vi "Identify.vi"(8 "error in (no error)":errorcluster, 11 "NI Generic Parser in":refnum<class "NI Generic Parser.lvclass">) -> (0 "error out":errorcluster, 2 "Plugin is Valid":bool, 3 "NI Generic Parser out":refnum<class "NI Generic Parser.lvclass">)   [LabVIEW 2016, in "NI Generic Parser.lvlib" / "NI Generic Parser.lvclass"]
uses:
  NI Generic Parser.lvclass
  C:/Sequence Automation/Plugins/File Parsing Interface.lvlibp/File Parsing Interface.lvclass
  Plugins/File Parsing Interface.lvlibp/Accessors/File to Parse/Read File to Parse.vi
  <vilib>/addons/_office/excel.llb/Excel Get Data ([str]).vi
  <vilib>/Utility/NIReport.llb/NI_report.lvclass
  <vilib>/Utility/NIReport.llb/Excel/NI_Excel.lvclass
  <vilib>/addons/_office/NI_ReportGenerationToolkit.lvlib
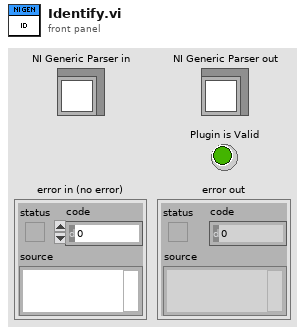
[diagram p1: front panel]
types:
  T1 = enum16{"Standard Report", "HTML", "Word", "Excel"}
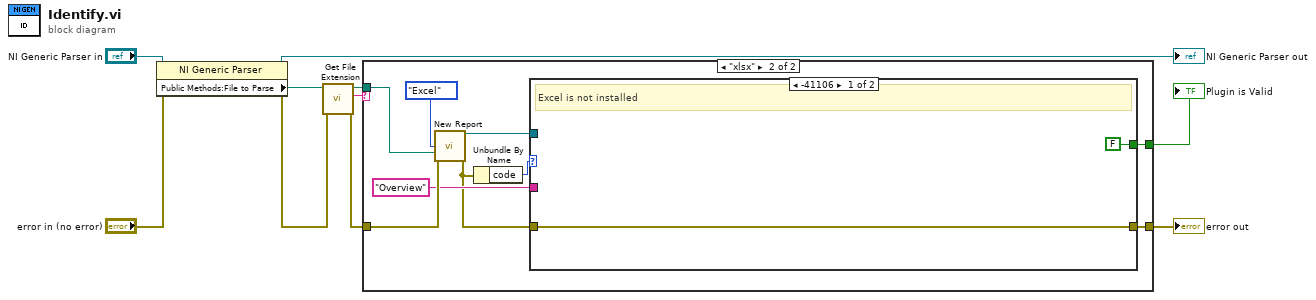
[diagram p0: block diagram]
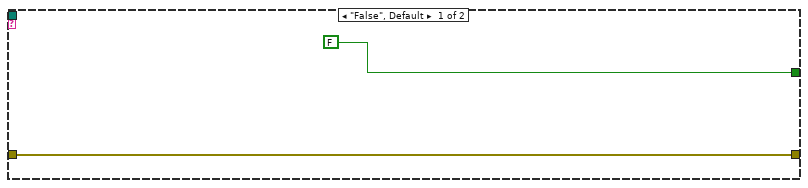
[diagram p2: hidden frame]
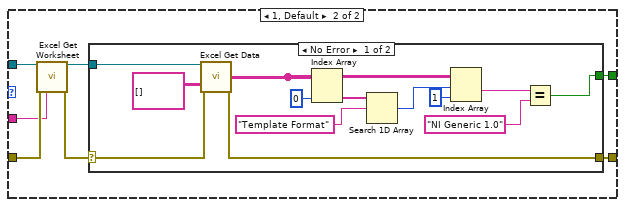
[diagram p3: hidden frame]
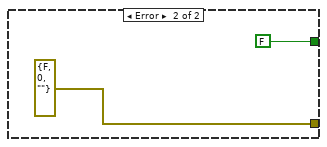
[diagram p4: hidden frame]
diagram:
  n1 = property class="NI Generic Parser"(reference="NI Generic Parser in", error in="error in (no error)") -> (reference out=→"NI Generic Parser out":refnum<class "NI Generic Parser.lvclass">, error out=w7:errorcluster, "Public Methods:File to Parse"=w6:path)
  n2 = call <vilib>:"Get File Extension.vi"("error in (no error)"=w7, "file"=w6) -> ("error out"=w4:errorcluster, "lowercase file extension"=w5:string, "dup file"=w2:path)  [unwired: 5 in, 2 out]
  n3 = case shown="\"xlsx\"" w5 {
    tunnel: w4 -> [w11 w19]
    tunnel: [FALSE w15] -> w3
    tunnel: w2 -> [_ w21]
    tunnel: [w11 w16] -> w1
    frame "False", Default {
    }
    frame "xlsx" {
      n4 = call <vilib>:"New Report.vi"("report type"=T1."Excel", "template (empty)"=w21, "error in (no error)"=w19) -> ("report out"=w18:refnum<class "NI_report.lvclass">, "error out"=w14:errorcluster)  [unwired: 11 in]
      n5 = Unbundle By Name(w14) -> ("code"=w13:i32)
      n6 = case shown="-41106" w13 {
        tunnel: w18 -> [_ w30]
        tunnel: w14 -> [w23 w29]
        tunnel: "Overview" ("name (\"\")") -> [_ w28]
        tunnel: [w23 w25] -> w16
        tunnel: [FALSE w24] -> w15
        frame -41106 {
          # "Excel is not installed"
        }
        frame 1, Default {
          n7 = call <vilib>:"Excel Get Worksheet.vi"("report in"=w30, "error in (no error)"=w29, "name (\"\")"=w28) -> ("report out"=w27:refnum<class "NI_report.lvclass">, "error out"=w26:errorcluster)  [unwired: 11 in]
          n8 = case shown="No Error" w26 {
            selector: w26 -> [w42 _]
            tunnel: w27 -> [w43 _]
            tunnel: [w40 errorcluster {"status"=FALSE, "code"=0, "source"=""} ("error out")] -> w25
            tunnel: [w31 FALSE] -> w24
            frame No Error {
              n9 = call-poly <vilib>:"Excel Get Data.vi"("report in"=w43, "data type"=string[][] [], "error in (no error)"=w42) -> ("data"=w36:string[][], "error out"=w40:errorcluster)  [unwired: 10 in, 1 out]
              n10 = Index Array(array=w36, index (col)=0 ("disabled index (col)")) -> (element=w38:string[])  [unwired: 1 in]
              n11 = Search 1D Array(1D array=w38, element="Template Format") -> (index of element=w35:i32)  [unwired: 1 in]
              n12 = Index Array(array=w36, index (row)=w35, index (col)=1 ("disabled index (col)")) -> (element=w33:string)
              n13 = Equal?(x=w33, y="NI Generic 1.0") -> (x = y?=w31:bool)
            }
            frame Error {
            }
          }
        }
      }
    }
  }
  "error out" <- w1
  "Plugin is Valid" <- w3
